vi "Build Result.vi"(9 "External Result Ref":string, 10 "Summary":string, 11 "Outcome":T1) -> (3 "Test Run Result":refnum<class "Test Run Result.lvclass">)   [LabVIEW 2026, in "Generic Execution Adapter.lvclass"]
uses:
  Generic Execution Adapter.lvclass
  Generic Execution Adapter.lvclass/Generic Execution Adapter.ctl
  Domain/Test Run Result/Test Run Result.lvclass
  Typedefs/enums/Run Outcome Enum.ctl
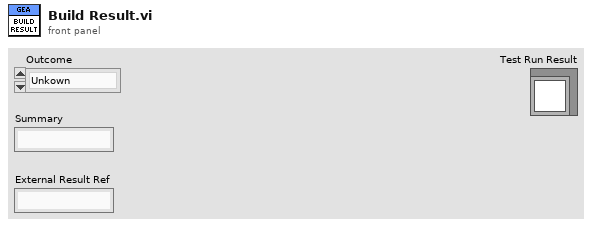
[diagram p1: front panel]
types:
  T1 = typedef "Run Outcome Enum.ctl" = enum16{"Unkown", "Passed", "Failed", "Error", "Aborted"}
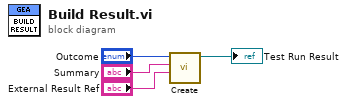
[diagram p0: block diagram]
diagram:
  n1 = call "Create.vi"("External Result Ref"="External Result Ref", "Summary"="Summary", "Outcome"="Outcome") -> ("Test Run Result"=→"Test Run Result":refnum<class "Test Run Result.lvclass">)  [unwired: 8 in]
